vi "indexSectionFromTable.vi"(9 "rowNum":i32, 10 "indexSec":string, 11 "tbl":string[][](array[string])) -> (3 "found?":bool)   [LabVIEW 2010]
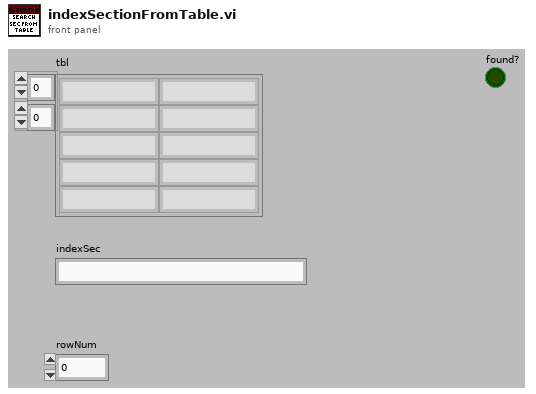
[diagram p1: front panel]
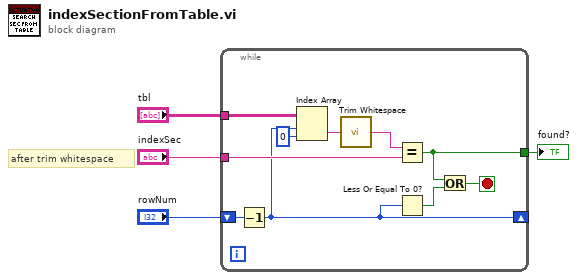
[diagram p0: block diagram]
diagram:
  # "after trim whitespace"
  n1 = while {
    shift-right: [w5] -> _
    shift-left: "rowNum" -> [w6]
    tunnel: "tbl" -> [w14]
    tunnel: "indexSec" -> [w8]
    tunnel: [w7] -> w1
    stop <- w10 stop-if-true
    n2 = Decrement(x=w6) -> (x-1=w5:i32)
    n3 = Index Array(array=w14, index (row)=w5, index (col)=0 ("disabled index (col)")) -> (element=w12:string)
    n4 = call <vilib>:"Trim Whitespace.vi"("string"=w12) -> ("trimmed string"=w9:string)  [unwired: 1 in]
    n5 = Equal?(x=w9, y=w8) -> (x = y?=w7:bool)
    n6 = Less Or Equal To 0?(x=w5) -> (x <= 0?=w11:bool)
    n7 = Or(x=w7, y=w11) -> (x .or. y?=w10:bool)
  }
  "found?" <- w1
